vi "CHROMA Set Frequency.vi"(8 "Error In":errorcluster, 10 "Frequency":dbl=60.0 min=15.0 max=1200.0, 11 "CHROMA VISA In":refnum<visa-resource-name>) -> (0 "Error Out":errorcluster, 3 "CHROMA VISA Out":refnum<visa-resource-name>)   [LabVIEW 2020]
uses:
  Type Definition/CHROMA Build CMD Type.ctl
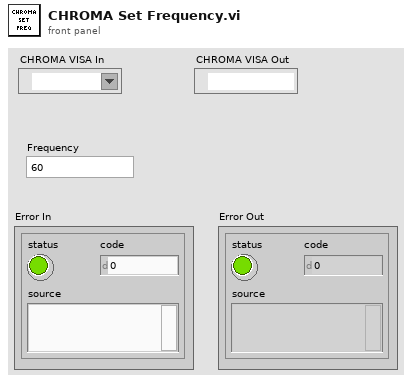
[diagram p1: front panel]
types:
  T1 = typedef "CHROMA Build CMD Type.ctl" = enum16{"Value DBL", "Value I32", "String"}
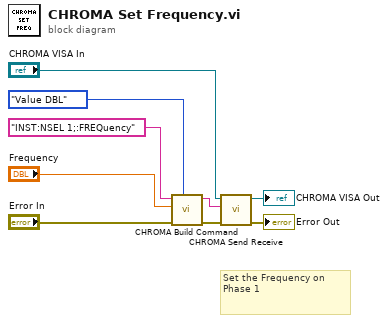
[diagram p0: block diagram]
diagram:
  # "Set the Frequency on Phase 1"
  n1 = call "CHROMA Build Command.vi"("Build Type"=CHROMA_Build_CMD_Type."Value DBL", "Error In"="Error In", "Value"="Frequency", "Partial Command"="INST:NSEL 1;:FREQuency" ("string to write")) -> ("Error Out"=w5:errorcluster, "Chroma Command"=w1:string)  [unwired: 6 in]
  n2 = call "CHROMA Send Receive.vi"("error in (no error)"=w5, "Send Command"=w1, "CHROMA VISA In"="CHROMA VISA In") -> ("error out"=→"Error Out":errorcluster, "CHROMA VISA Out"=→"CHROMA VISA Out":refnum<visa-resource-name>)  [unwired: 6 in, 1 out]
